vi "子界面.vi"() -> ()   [LabVIEW 2018]
panel:
  in  "数值":dbl
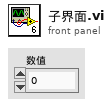
[diagram p1: front panel]
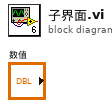
[diagram p0: block diagram]
diagram:
